vi "seti_labview_read_parameters_from_file.vi"(8 "error in (no error)":errorcluster) -> (0 "error out":errorcluster, 1 "start_icfft":i32, 2 "Chirp FFT Pairs":T2[](array[typedef]), 3 "binWorkUnitDataPoints.bin (DataIn)":csg[](array[numeric]), 4 "Array of Power Spectrum Data":T1[](array[typedef]), 5 "NumDataPoints":u32, 7 "end_icfft":i32)   [LabVIEW 2014, in "SETI_LV.lvlib"]
uses:
  SETI_LV/SETI_LV.lvlib
  ChirpFFT Pairs.ctl
  Power Spectrum Data.ctl
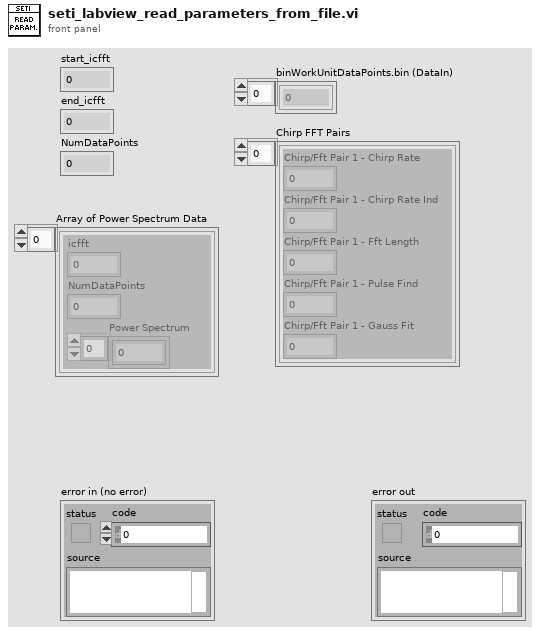
[diagram p1: front panel]
types:
  T1 = typedef "SETI_LV.lvlib/Power Spectrum Data.ctl" = cluster{"icfft":i32, "NumDataPoints":i32, "Power Spectrum":sgl[]}
  T2 = typedef "SETI_LV.lvlib/ChirpFFT Pairs.ctl" = cluster{"Chirp/Fft Pair 1 - Chirp Rate":dbl, "Chirp/Fft Pair 1 - Chirp Rate Ind":i32, "Chirp/Fft Pair 1 - Fft Length":i32, "Chirp/Fft Pair 1 - Pulse Find":i32, "Chirp/Fft Pair 1 - Gauss Fit":i32}
  T3 = enum16{"big-endian, network order", "native, host order", "little-endian"}
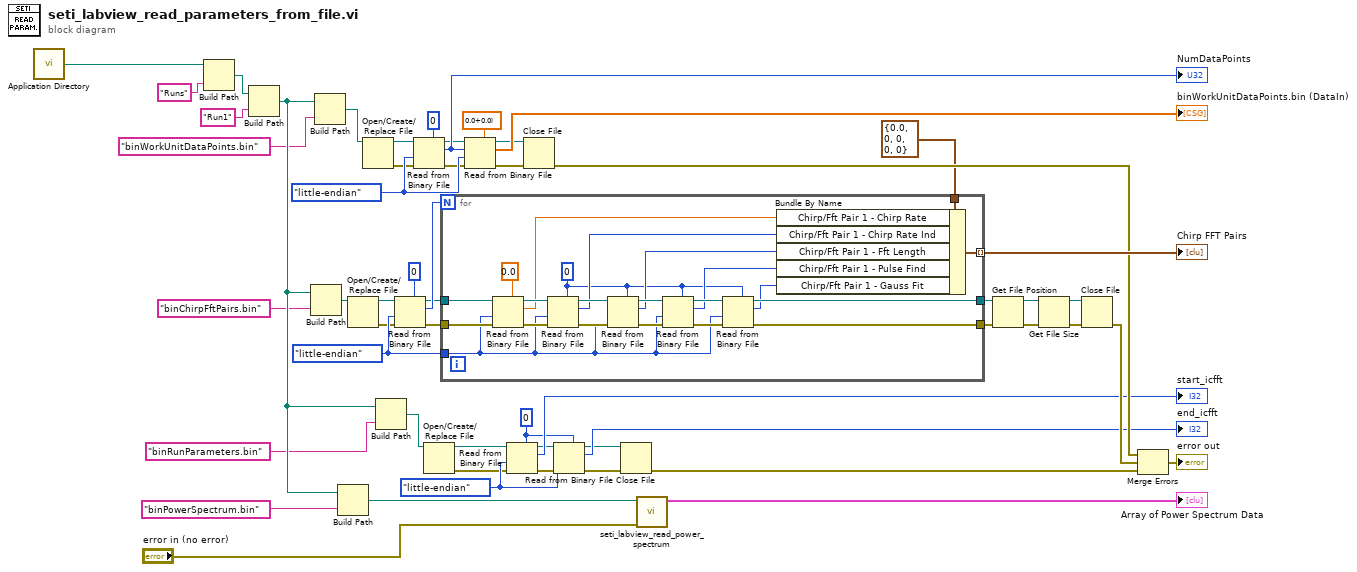
[diagram p0: block diagram]
diagram:
  w32 = T3."little-endian" ("byte order (0:big-endian, network order)")
  w38 = 0
  w17 = T3."little-endian" ("byte order (0:big-endian, network order)")
  w37 = T3."little-endian" ("byte order (0:big-endian, network order)")
  n1 = call <vilib>:"Application Directory.vi"() -> ("Application Directory"=w1:path)
  n2 = Build Path(base path=w1, name or relative path="Runs") -> (appended path=w46:path)
  n3 = Build Path(base path=w46, name or relative path="Run1") -> (appended path=w48:path)
  n4 = Build Path(base path=w48, name or relative path="binChirpFftPairs.bin") -> (appended path=w10:path)
  n5 = Build Path(base path=w48, name or relative path="binWorkUnitDataPoints.bin") -> (appended path=w8:path)
  n6 = Build Path(base path=w48, name or relative path="binPowerSpectrum.bin") -> (appended path=w41:path)
  n7 = Open/Create/Replace File(file path (use dialog)=w10) -> (refnum out=w15:refnum<file>, error out=w14:errorcluster)  [unwired: 5 in, 1 out]
  n8 = Open/Create/Replace File(file path (use dialog)=w8) -> (refnum out=w2:refnum<file>, error out=w3:errorcluster)  [unwired: 5 in, 1 out]
  n9 = Build Path(base path=w48, name or relative path="binRunParameters.bin") -> (appended path=w29:path)
  n10 = Read from Binary File(5:0, 8:w14, 9:w17, 11:w15) -> (0:w16:errorcluster, 2:w18:i32, 3:w12:refnum<file>)  [unwired: 2 in, 1 out]
  n11 = Read from Binary File(5:u32 0, 8:w3, 9:w37, 11:w2) -> (0:w35:errorcluster, 2:w42:u32, 3:w6:refnum<file>)  [unwired: 2 in, 1 out]
  "NumDataPoints" <- w42
  n12 = Open/Create/Replace File(file path (use dialog)=w29) -> (refnum out=w26:refnum<file>, error out=w27:errorcluster)  [unwired: 5 in, 1 out]
  n13 = for {
    N: w18 -> [_]
    tunnel: w12 -> [w76]
    tunnel: w16 -> [w75]
    tunnel: w17 -> [w66]
    tunnel: [w65] -> w20
    tunnel: [w64] -> w21
    tunnel: T2 {"Chirp/Fft Pair 1 - Chirp Rate"=0.0, "Chirp/Fft Pair 1 - Chirp Rate Ind"=0, "Chirp/Fft Pair 1 - Fft Length"=0, "Chirp/Fft Pair 1 - Pulse Find"=0, "Chirp/Fft Pair 1 - Gauss Fit"=0} ("Chirp/Fft Pairs") -> [w63]
    tunnel: [w57] -> w54 mode=indexing
    w56 = 0
    n14 = Read from Binary File(5:0.0, 8:w75, 9:w66, 11:w76) -> (0:w73:errorcluster, 2:w62:dbl, 3:w74:refnum<file>)  [unwired: 2 in, 1 out]
    n15 = Read from Binary File(5:w56, 8:w73, 9:w66, 11:w74) -> (0:w71:errorcluster, 2:w61:i32, 3:w72:refnum<file>)  [unwired: 2 in, 1 out]
    n16 = Read from Binary File(5:w56, 8:w71, 9:w66, 11:w72) -> (0:w67:errorcluster, 2:w60:i32, 3:w68:refnum<file>)  [unwired: 2 in, 1 out]
    n17 = Read from Binary File(5:w56, 8:w67, 9:w66, 11:w68) -> (0:w70:errorcluster, 2:w59:i32, 3:w69:refnum<file>)  [unwired: 2 in, 1 out]
    n18 = Read from Binary File(5:w56, 8:w70, 9:w66, 11:w69) -> (0:w64:errorcluster, 2:w58:i32, 3:w65:refnum<file>)  [unwired: 2 in, 1 out]
    n19 = Bundle By Name(cluster=w63, "Chirp/Fft Pair 1 - Chirp Rate"=w62, "Chirp/Fft Pair 1 - Chirp Rate Ind"=w61, "Chirp/Fft Pair 1 - Fft Length"=w60, "Chirp/Fft Pair 1 - Pulse Find"=w59, "Chirp/Fft Pair 1 - Gauss Fit"=w58) -> (w57:T2)
  }
  "Chirp FFT Pairs" <- w54
  n20 = Read from Binary File(5:csg 0.0+0.0i, 8:w35, 9:w37, 10:w42, 11:w6) -> (0:w36:errorcluster, 2:→"binWorkUnitDataPoints.bin (DataIn)":csg[], 3:w5:refnum<file>)  [unwired: 1 in, 1 out]
  n21 = Read from Binary File(5:w38, 8:w27, 9:w32, 11:w26) -> (0:w31:errorcluster, 2:→"start_icfft":i32, 3:w30:refnum<file>)  [unwired: 2 in, 1 out]
  n22 = Close File(refnum=w5, error in=w36) -> (error out=w51:errorcluster)  [unwired: 1 out]
  n23 = Read from Binary File(5:w38, 8:w31, 9:w32, 11:w30) -> (0:w34:errorcluster, 2:→"end_icfft":i32, 3:w33:refnum<file>)  [unwired: 2 in, 1 out]
  n24 = Close File(refnum=w33, error in=w34) -> (error out=w49:errorcluster)  [unwired: 1 out]
  n25 = call "seti_labview_read_power_spectrum.vi"("error in (no error)"="error in (no error)", "Power Spectrum Data file path"=w41) -> ("Array of Power Spectrum Data"=→"Array of Power Spectrum Data":T1[])  [unwired: 8 in, 1 out]
  n26 = Get File Position(4:w21, 7:w20) -> (0:w22:errorcluster, 3:w23:refnum<file>)  [unwired: 1 out]
  n27 = Get File Size(file=w23, error in=w22) -> (refnum out=w24:refnum<file>, 0:w25:errorcluster)  [unwired: 1 out]
  n28 = Close File(refnum=w24, error in=w25) -> (error out=w50:errorcluster)  [unwired: 1 out]
  n29 = Merge Errors(w51, w50, w49) -> (→"error out":errorcluster)
